vi "RunDuringExperiment1.vi"(8 "Error In":errorcluster, 10 "Params":T1={"Restarted"=FALSE, "Enable Calibration"=FALSE, "Position Shift Limit (Microns)"=3.0, "Frame Num"=0.0, "Sampling Interval"=0.0, "Analyze Nth Frames"=1}, 11 "Motion Data In":T3) -> (0 "Error Out":errorcluster, 1 "Motion Computation Error":errorcluster, 3 "Shifts Out":T2)   [LabVIEW 2014]
uses:
  GlobalVars.vi
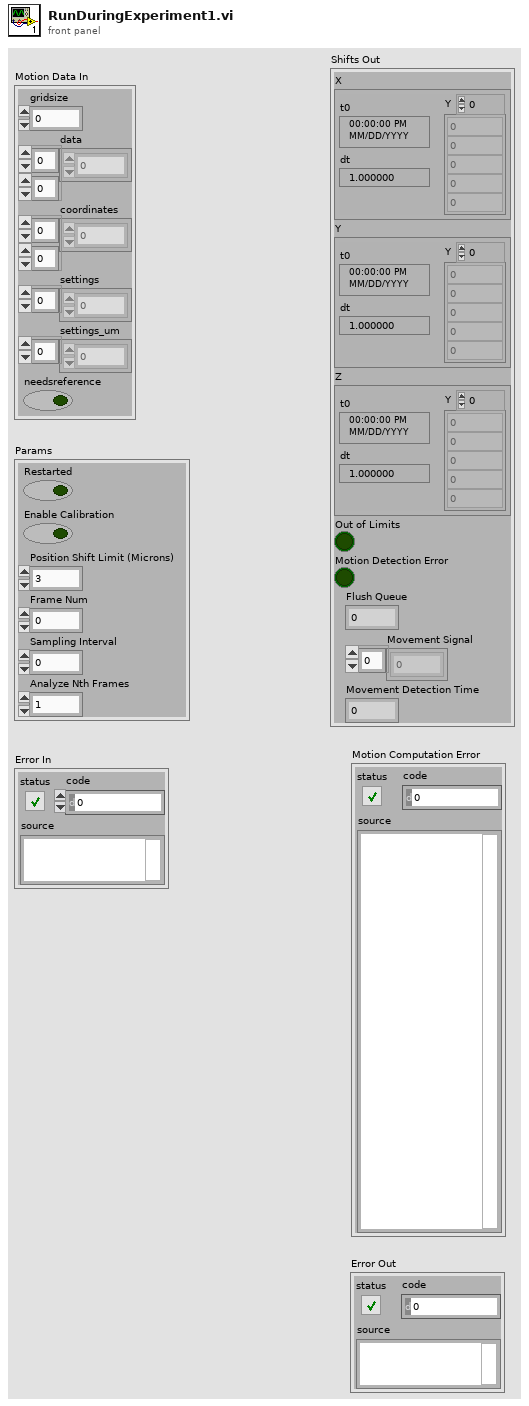
[diagram p1: front panel]
types:
  T1 = cluster{"Restarted":bool, "Enable Calibration":bool, "Position Shift Limit (Microns)":dbl, "Frame Num":dbl, "Sampling Interval":dbl, "Analyze Nth Frames":i32}
  T2 = cluster{"X":waveform(dbl), "Y":waveform(dbl), "Z":waveform(dbl), "Out of Limits":bool, "Motion Detection Error":bool, "Flush Queue":i32, "Movement Signal":dbl[], "Movement Detection Time":dbl}
  T3 = cluster{"gridsize":u16, "data":i32[][], "coordinates":i32[][], "settings":i32[], "settings_um":i32[], "needsreference":bool}
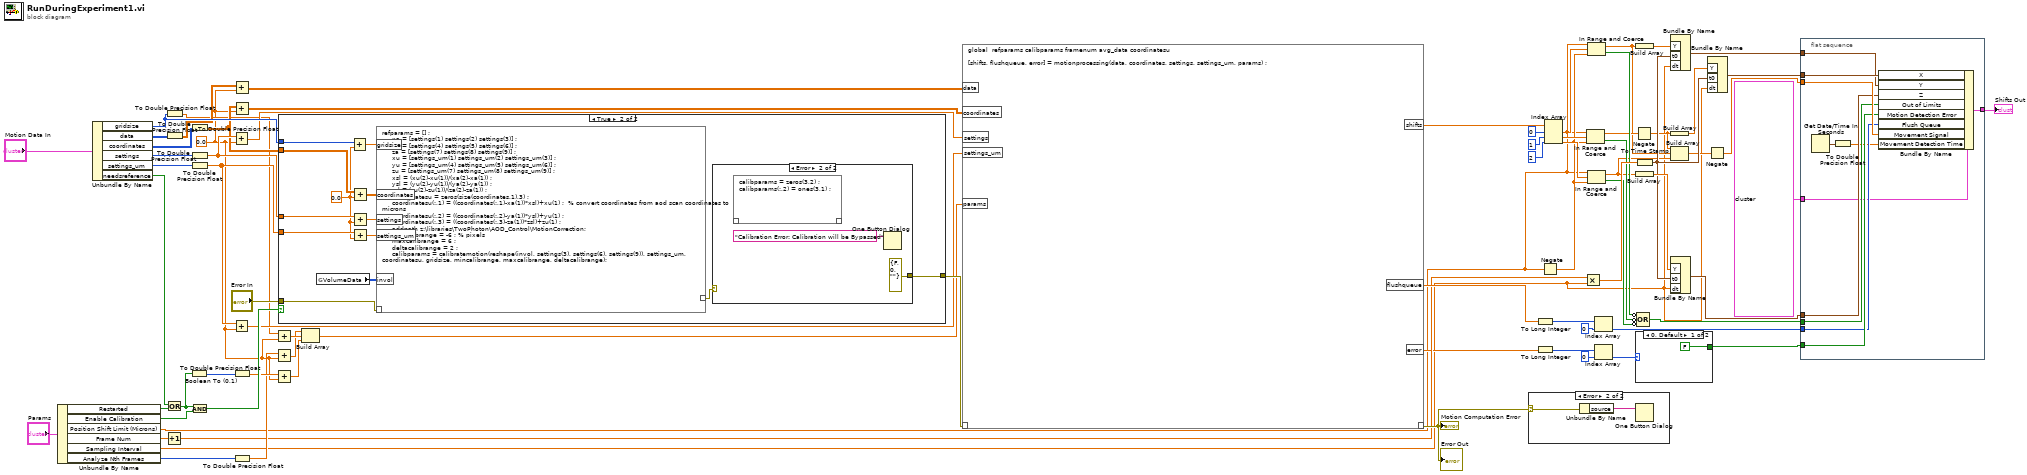
[diagram p0: block diagram]
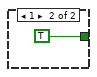
[diagram p2: hidden frame]
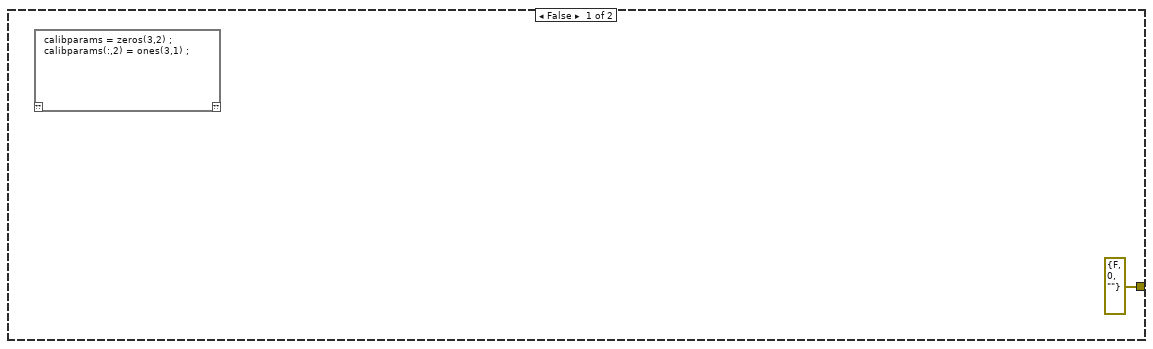
[diagram p4: hidden frame]
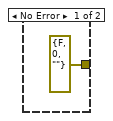
[diagram p5: hidden frame]
diagram:
  w50 = 0.0 ("y")
  n1 = Unbundle By Name("Params") -> ("Restarted"=w6:bool, "Enable Calibration"=w5:bool, "Position Shift Limit (Microns)"=w4:dbl, "Frame Num"=w3:dbl, "Sampling Interval"=w2:dbl, "Analyze Nth Frames"=w1:i32)
  n2 = Unbundle By Name("Motion Data In") -> ("gridsize"=w64:u16, "data"=w70:i32[][], "coordinates"=w69:i32[][], "settings"=w68:i32[], "settings_um"=w67:i32[], "needsreference"=w49:bool)
  n3 = Or(x=w49, y=w6) -> (x .or. y?=w48:bool)
  n4 = Increment(x=w3) -> (x+1=w43:dbl)
  n5 = To Double Precision Float(number=w64) -> (double precision float=w52:dbl)
  n6 = To Double Precision Float(number=w70) -> (double precision float=w54:dbl[][])
  n7 = Boolean To (0,1)(Boolean=w48) -> (0, 1=w66:i16)
  n8 = To Double Precision Float(number=w69) -> (double precision float=w56:dbl[][])
  n9 = To Double Precision Float(number=w68) -> (double precision float=w58:dbl[])
  n10 = To Double Precision Float(number=w67) -> (double precision float=w60:dbl[])
  n11 = And(x=w48, y=w5) -> (x .and. y?=w63:bool)
  n12 = Add(x=w58, y=w50) -> (x+y=w57:dbl[])
  n13 = Add(x=w60, y=w50) -> (x+y=w59:dbl[])
  n14 = Add(x=w54, y=w50) -> (x+y=w53:dbl[][])
  n15 = Add(x=w56, y=w50) -> (x+y=w55:dbl[][])
  n16 = To Double Precision Float(number=w66) -> (double precision float=w61:dbl)
  n17 = To Double Precision Float(number=w1) -> (double precision float=w51:dbl)
  n18 = Add(x=w52, y=w50) -> (x+y=w45:dbl)
  n19 = Add(x=w51, y=w50) -> (x+y=w44:dbl)
  n20 = Add(x=w61, y=w50) -> (x+y=w47:dbl)
  n21 = case shown="True" w63 {
    tunnel: w64 -> [_ w79]
    tunnel: w56 -> [_ w81]
    tunnel: w58 -> [_ w83]
    tunnel: w60 -> [_ w85]
    tunnel: [errorcluster {"status"=FALSE, "code"=0, "source"=""} ("error IO") w86] -> w62
    tunnel: "Error In" -> [_ w76]
    frame False {
      n22 = script code="calibparams = zeros(3,2) ;\ncalibparams(:,2) = ones(3,1) ;"() -> ()  [unwired: 1 in, 1 out]
    }
    frame True {
      w78 = 0.0 ("y")
      n23 = global read "GlobalVars.vi" "VolumeData"() -> (w88:i32[][])
      n24 = Add(x=w79, y=w78) -> (x+y=w77:dbl)
      n25 = Add(x=w81, y=w78) -> (x+y=w80:dbl[][])
      n26 = Add(x=w83, y=w78) -> (x+y=w82:dbl[])
      n27 = Add(x=w85, y=w78) -> (x+y=w84:dbl[])
      n28 = script code="refparams = [] ;\n     xa = [settings(1) settings(2) settings(3)] ;\n     ya = [settings(4) settings(5) settings(6)] ;\n     za = [settings(7) settings(8) settings(9)] ;\n     xu = [settings_um(1) settings_um(2) settings_um(3)] ;\n     yu = [settings_um(4) settings_um(5) settings_um(6)] ;\n     zu = [settings_um(7) settings_um(8) settings_um(9)] ;\n     xsl = (xu(2)-xu(1))/(xa(2)-xa(1)) ;\n     ysl = (yu(2)-yu(1))/(ya(2)-ya(1)) ;\n     zsl = (zu(2)-zu(1))/(za(2)-za(1)) ;\n     coordinatesu = zeros(size(coordinates,1),3) ;\n     coordinatesu(:,1) = ((coordinates(:,1)-xa(1))*xsl)+xu(1) ;  % convert coordinates from aod scan coordinates to microns\n     coordinatesu(:,2) = ((coordinates(:,2)-ya(1))*ysl)+yu(1) ;\n     coordinatesu(:,3) = ((coordinates(:,3)-za(1))*zsl)+zu(1) ;\n     addpath z:\\libraries\\TwoPhoton\\AOD_Control\\MotionCorrection;\n     mincalibrange = -6 ; % pixels\n     maxcalibrange = 6 ;\n     deltacalibrange = 2 ;\n     calibparams = calibratemotion(reshape(invol, settings(3), settings(6), settings(9)), settings_um, coordinatesu, gridsize, mincalibrange, maxcalibrange, deltacalibrange);"("??"=w76, "coordinates"=w80, "gridsize"=w77, "settings"=w82, "settings_um"=w84, "invol"=w88) -> ("??"=w87:errorcluster)
      n29 = case shown="Error" w87 {
        tunnel: [errorcluster {"status"=FALSE, "code"=0, "source"=""} ("error IO") errorcluster {"status"=FALSE, "code"=0, "source"=""} ("error IO")] -> w86
        frame No Error {
        }
        frame Error {
          n30 = script code="calibparams = zeros(3,2) ;\ncalibparams(:,2) = ones(3,1) ;"() -> ()  [unwired: 1 in, 1 out]
          n31 = One Button Dialog(message="Calibration Error: Calibration will be Bypassed") -> ()  [unwired: 1 in, 1 out]
        }
      }
    }
  }
  n32 = Build Array(w44, w45, w47) -> (w46:dbl[])
  n33 = script code="global  refparams calibparams framenum avg_data coordinatesu\n\n[shifts, flushqueue, error] = motionprocessing(data, coordinates, settings, settings_um, params) ;"("??"=w62, "data"=w53, "coordinates"=w55, "settings"=w57, "settings_um"=w59, "params"=w46) -> ("??"=w74:errorcluster, "shifts"=w71:dbl[], "flushqueue"=w65:dbl[], "error"=w42:dbl[])
  "Error Out" <- w74
  "Motion Computation Error" <- w74
  n34 = case shown="Error" w74 {
    selector: w74 -> [_ w93]
    frame No Error {
    }
    frame Error {
      n35 = Unbundle By Name(w93) -> ("source"=w92:string)
      n36 = One Button Dialog(message=w92) -> ()  [unwired: 1 in, 1 out]
    }
  }
  n37 = To Long Integer(number=w65) -> (32bit integer=w41:i32[])
  n38 = To Long Integer(number=w42) -> (32bit integer=w39:i32[])
  n39 = Negate(x=w4) -> (-x=w17:dbl)
  n40 = Index Array(array=w71, index #1=0 ("index"), index #2=1 ("index"), index #3=2 ("index")) -> (element #1=w31:dbl, element #2=w30:dbl, element #3=w29:dbl)
  n41 = Multiply(x=w43, y=w2) -> (x*y=w33:dbl)
  n42 = In Range and Coerce(upper limit=w4, x=w30, lower limit=w17) -> (coerced(x)=w21:dbl, In Range?=w27:bool)
  n43 = In Range and Coerce(upper limit=w4, x=w31, lower limit=w17) -> (coerced(x)=w19:dbl, In Range?=w28:bool)
  n44 = In Range and Coerce(upper limit=w4, x=w29, lower limit=w17) -> (coerced(x)=w25:dbl, In Range?=w26:bool)
  n45 = Index Array(array=w41, index=0 ("index (row)")) -> (element=w10:i32)
  n46 = Index Array(array=w39, index=0) -> (element=w37:i32)
  n47 = Build Array(w19) -> (w34:dbl[])
  n48 = Negate(x=w21) -> (-x=w20:dbl)
  n49 = Build Array(w25) -> (w35:dbl[])
  n50 = case shown="0, Default" w37 {
    tunnel: [FALSE ("Motion Detection Error") TRUE ("Motion Detection Error")] -> w11
    frame 0, Default {
    }
    frame 1 {
    }
  }
  n51 = To Time Stamp(1:w33) -> (0:w32:timestamp)
  n52 = Compound Arithmetic op=OR(invert w28, invert w27, invert w26) -> (w12:bool)
  n53 = Bundle By Name("Y"=w34, "t0"=w32, "dt"=w2) -> (w14:waveform(dbl))  [unwired: 1 in]
  n54 = Bundle By Name("Y"=w35, "t0"=w32, "dt"=w2) -> (w13:waveform(dbl))  [unwired: 1 in]
  n55 = Build Array(w20) -> (w36:dbl[])
  n56 = Build Array(w20, w19, w25) -> (w18:dbl[])
  n57 = Bundle By Name("Y"=w36, "t0"=w32, "dt"=w2) -> (w15:waveform(dbl))  [unwired: 1 in]
  n58 = Negate(x=w18) -> (-x=w16:dbl[])
  n59 = flat-sequence {
    tunnel: w16 -> [w106]
    tunnel: w15 -> [w105]
    tunnel: w14 -> [w104]
    tunnel: w13 -> [w103]
    tunnel: w12 -> [w102]
    tunnel: w11 -> [w101]
    tunnel: w10 -> [w100]
    tunnel: T2 {"X"={"t0"=timestamp(0 s since 1904-01-01), "dt"=1.0, "Y"=[]}, "Y"={"t0"=timestamp(0 s since 1904-01-01), "dt"=1.0, "Y"=[]}, "Z"={"t0"=timestamp(0 s since 1904-01-01), "dt"=1.0, "Y"=[]}, "Out of Limits"=FALSE, "Motion Detection Error"=FALSE, "Flush Queue"=0, "Movement Signal"=[], "Movement Detection Time"=0.0} ("Cluster") -> [w99]
    tunnel: [w98] -> w8
    frame #0 {
      n60 = Get Date/Time In Seconds() -> (seconds since 1Jan1904=w97:timestamp)
      n61 = To Double Precision Float(number=w97) -> (double precision float=w96:dbl)
      n62 = Bundle By Name(cluster=w99, "X"=w105, "Y"=w104, "Z"=w103, "Out of Limits"=w102, "Motion Detection Error"=w101, "Flush Queue"=w100, "Movement Signal"=w106, "Movement Detection Time"=w96) -> (w98:T2)
    }
  }
  "Shifts Out" <- w8
